vi "Generate Error.vi"(6 "Include Call Chain? (False)":bool, 7 "Status (True)":bool=TRUE, 8 "error in":errorcluster, 10 "Error Input Values":variant, 11 "Error Code":i32) -> (0 "Generated Error":errorcluster)   [LabVIEW 2021]
doc: "Generate error with specific <b>Error Code</b> from the list of error codes specified in <b>*erros.xml</b> file. \nIf the error has a parametric description, wire the parameter values into <b>Error Input Values</b> preferably as a cluster of values or an array (in case of multiple inputs) in the same order, as they are stated in the error description. To format error messages use the same syntax as you would use in the Format Into String function.\n<b>Status (True)</b> set to True to report that an <b>error</b> occurred, set to False to signal a <b>warning</b>\n<b>Include Call Chain? (False)</b> appends the call chain of the VI where the error occurred at the end of the error description.\nError with specific code and source message is outputed at <b>Generated Error</b> output."
uses:
  <vilib>/Utility/error.llb/whitespace.ctl
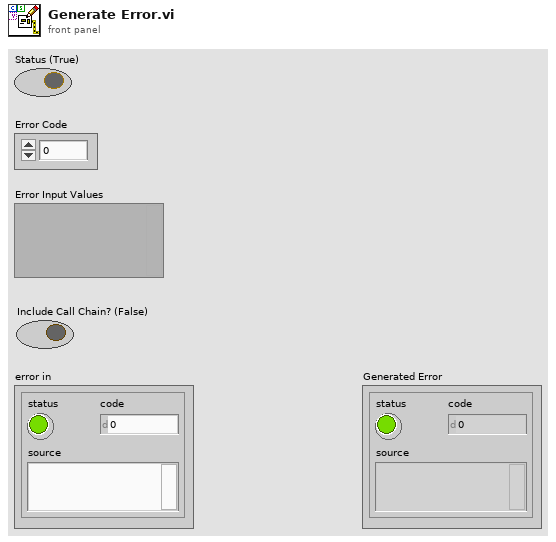
[diagram p1: front panel]
types:
  T1 = typedef "whitespace.ctl" = u16
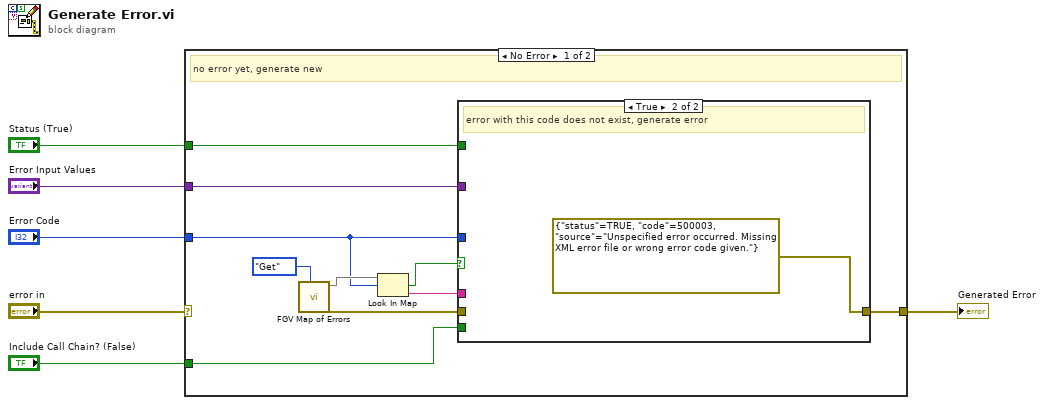
[diagram p0: block diagram]
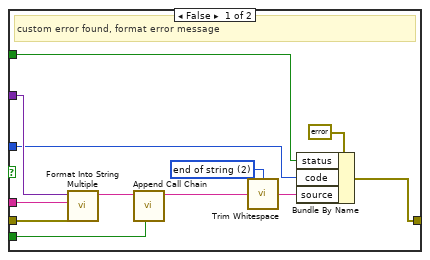
[diagram p2: hidden frame]
diagram:
  n1 = case shown="No Error" "error in" {
    selector: "error in" -> [_ w30]
    tunnel: [w16 w30] -> w6
    tunnel: "Error Input Values" -> [w15 _]
    tunnel: "Error Code" -> [w10 _]
    tunnel: "Include Call Chain? (False)" -> [w8 _]
    tunnel: "Status (True)" -> [w7 _]
    frame No Error {
      # "no error yet, generate new"
      n2 = call "FGV Map of Errors.vi"("Operation (Get)"=enum16{"Init", "Get", "Update"}."Get") -> ("error out"=w9:errorcluster, "Custom Errors out"=w13:map{i32, string})  [unwired: 9 in]
      n3 = Look In Map(map=w13, key=w10) -> (key not found?=w12:bool, value=w11:string)  [unwired: 1 in]
      n4 = case shown="True" w12 {
        tunnel: w9 -> [w26 _]
        tunnel: [w23 errorcluster {"status"=TRUE, "code"=500003, "source"="Unspecified error occurred. Missing XML error file or wrong error code given."} ("error IO")] -> w16
        tunnel: w11 -> [w27 _]
        tunnel: w15 -> [w28 _]
        tunnel: w10 -> [w24 _]
        tunnel: w8 -> [w21 _]
        tunnel: w7 -> [w20 _]
        frame False {
          w17 = T1 2 items=["both", "start of string", "end of string"] ("location (both)")
          # "custom error found, format error message"
          n5 = call "Format Into String Multiple.vi"("error in"=w26, "Format String"=w27, "Input Values"=w28) -> ("Formated String"=w22:string)  [unwired: 7 in, 1 out]
          n6 = call "Append Call Chain.vi"("Include Call Chain?"=w21, "Input String"=w22) -> ("Output String"=w19:string)  [unwired: 9 in]
          n7 = call <vilib>:"Trim Whitespace.vi"("string"=w19, "location (both)"=w17) -> ("trimmed string"=w18:string)
          n8 = Bundle By Name(cluster=errorcluster {"status"=FALSE, "code"=0, "source"=""} ("error constant"), "status"=w20, "code"=w24, "source"=w18) -> (w23:errorcluster)
        }
        frame True {
          # "error with this code does not exist, generate error"
        }
      }
    }
    frame Error {
      # "error already occurred, just forward it"
    }
  }
  "Generated Error" <- w6
